vi "Lidar Control Error.vi"(0 "Lidar Motor Control":T1={"Reset Encoder"=FALSE, "Motor Enable"=FALSE, "Choice of Control Type"=enum."Direct Voltage Control", "Choice of Oscillation"=enum."Oscillate Voltage", "Choice of Compensation"=enum."None", "Choice of Error"=enum."Gray Error", "Units of pi rad 18b (s-fxp-1)"={"Phi_B Set Point (pi rad)"=0.0, "Phi_A Set Point (pi rad)"=0.0, "Phi_Lidar Set Point (pi rad)"=0.0, "Phi_Lidar - Phi_A"=0.0, "Phi_mass-Phi_Lidar"=0.0, "Convert (enc) to (pi rad)"=0.0, "Oscillation Frequency (pi rad per 100KHz)"=0.0}, "Units of 18b (s-fxp-1) gain"={"Proportional Gain"=0.0, " Integral Gain"=0.0, "Oscillation Setpoint Amplitude"=0.0, "Gravity Compensation Gain"=0.0, "Phi_B Set Point (enc) pre-gain"=0.0, "Phi_B Set Point (pi rad) pre-gain"=0.0, "Phi_A Set Point (pi rad) pre-gain"=0.0, "Phi_Lidar Set Point (pi rad) pre-gain"=0.0, "Derivative Gain"=0.0, "Double Integral Gain"=0.0, "Second Derivative Gain"=0.0}, "Units of 20b s-fxp-5 Voltage"={"Oscillation Voltage Amplitude"=0.0, "Motor Voltage"=0.0}, "Units of encoder 32b uint"={"Phi_B Set Point (enc)"=0, "Lidar Encoder Cap"=0}, "Debug Args"=[FALSE, FALSE, FALSE, FALSE, FALSE, FALSE, FALSE, FALSE, FALSE, FALSE, FALSE, FALSE, FALSE, FALSE, FALSE, FALSE, FALSE, FALSE, FALSE, FALSE], "Units of 8b int gain exponents"={"Proportional Gain"=0, " Integral Gain"=0, "Oscillation Setpoint Amplitude"=0, "Gravity Compensation Gain"=0, "Phi_B Set Point (enc) pre-gain"=0, "Phi_B Set Point (pi rad) pre-gain"=0, "Phi_A Set Point (pi rad) pre-gain"=0, "Phi_Lidar Set Point (pi rad) pre-gain"=0, "Derivative Gain"=0, "Double Integral Gain"=0, "Second Derivative Gain"=0}, "6b (u-fxp-6)"={"Size of Integrator"=0.0, "Size of IIntigrator"=0.0, "Size of Differentiator"=0.0, "Size of DDifferentiator"=0.0}} {"Units of 20b s-fxp-5 Voltage"."Motor Voltage" format="%.17g"}) -> ()   [LabVIEW 2009]
uses:
  Strict Lidar Motor Control Cluster.ctl
  [Debug] Global.vi
  Motor Output Global.vi
  Motor Control Global.vi
panel:
  out "I Error":fxp<+/-,18,1> format="%.18g"
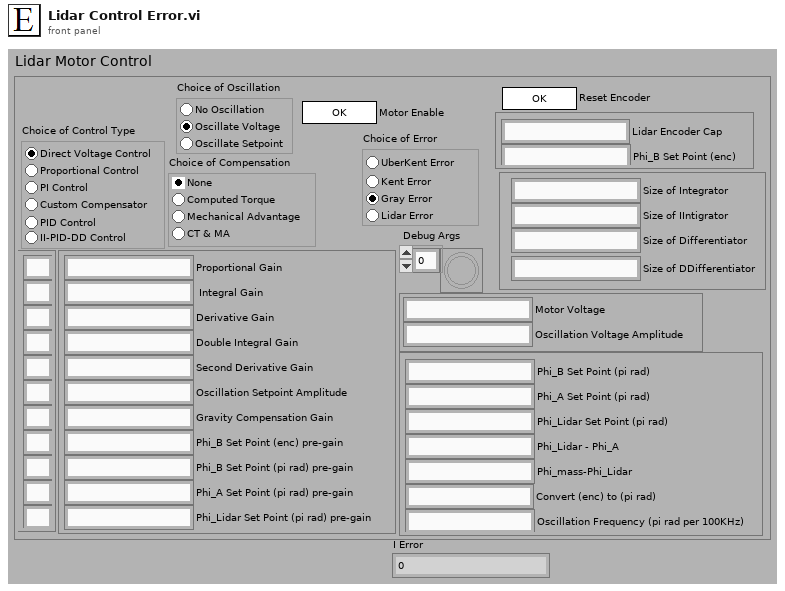
[diagram p1: front panel]
types:
  T1 = typedef "Strict Lidar Motor Control Cluster.ctl" = cluster{"Reset Encoder":bool, "Motor Enable":bool, "Choice of Control Type":enum32{"Direct Voltage Control", "Proportional Control", "PI Control", "Custom Compensator", "PID Control", "II-PID-DD Control"}, "Choice of Oscillation":enum32{"Oscillate Voltage", "Oscillate Setpoint", "No Oscillation"}, "Choice of Compensation":enum32{"None", "Computed Torque", "Mechanical Advantage", "CT & MA "}, "Choice of Error":enum32{"Gray Error", "Lidar Error", "Kent Error", "UberKent Error"}, "Units of pi rad 18b (s-fxp-1)":cluster{"Phi_B Set Point (pi rad)":fxp<+/-,18,1>, "Phi_A Set Point (pi rad)":fxp<+/-,18,1>, "Phi_Lidar Set Point (pi rad)":fxp<+/-,18,1>, "Phi_Lidar - Phi_A":fxp<+/-,18,1>, "Phi_mass-Phi_Lidar":fxp<+/-,18,1>, "Convert (enc) to (pi rad)":fxp<+/-,18,1>, "Oscillation Frequency (pi rad per 100KHz)":fxp<+/-,18,1>}, "Units of 18b (s-fxp-1) gain":cluster{"Proportional Gain":fxp<+/-,18,1>, " Integral Gain":fxp<+/-,18,1>, "Oscillation Setpoint Amplitude":fxp<+/-,18,1>, "Gravity Compensation Gain":fxp<+/-,18,1>, "Phi_B Set Point (enc) pre-gain":fxp<+/-,18,1>, "Phi_B Set Point (pi rad) pre-gain":fxp<+/-,18,1>, "Phi_A Set Point (pi rad) pre-gain":fxp<+/-,18,1>, "Phi_Lidar Set Point (pi rad) pre-gain":fxp<+/-,18,1>, "Derivative Gain":fxp<+/-,18,1>, "Double Integral Gain":fxp<+/-,18,1>, "Second Derivative Gain":fxp<+/-,18,1>}, "Units of 20b s-fxp-5 Voltage":cluster{"Oscillation Voltage Amplitude":fxp<+/-,20,5>, "Motor Voltage":fxp<+/-,20,5>}, "Units of encoder 32b uint":cluster{"Phi_B Set Point (enc)":i32, "Lidar Encoder Cap":i32}, "Debug Args":bool[], "Units of 8b int gain exponents":cluster{"Proportional Gain":i8, " Integral Gain":i8, "Oscillation Setpoint Amplitude":i8, "Gravity Compensation Gain":i8, "Phi_B Set Point (enc) pre-gain":i8, "Phi_B Set Point (pi rad) pre-gain":i8, "Phi_A Set Point (pi rad) pre-gain":i8, "Phi_Lidar Set Point (pi rad) pre-gain":i8, "Derivative Gain":i8, "Double Integral Gain":i8, "Second Derivative Gain":i8}, "6b (u-fxp-6)":cluster{"Size of Integrator":fxp<+,6,6>, "Size of IIntigrator":fxp<+,6,6>, "Size of Differentiator":fxp<+,6,6>, "Size of DDifferentiator":fxp<+,6,6>}}
  T2 = enum32{"Gray Error", "Lidar Error", "Kent Error", "UberKent Error"}
  T3 = cluster{"Debug Args[0]":bool, "Debug Args[1]":bool, "Debug Args[2]":bool, "Debug Args[3]":bool, "Debug Args[4]":bool, "Debug Args[5]":bool, "Debug Args[6]":bool, "Debug Args[7]":bool, "Debug Args[8]":bool}
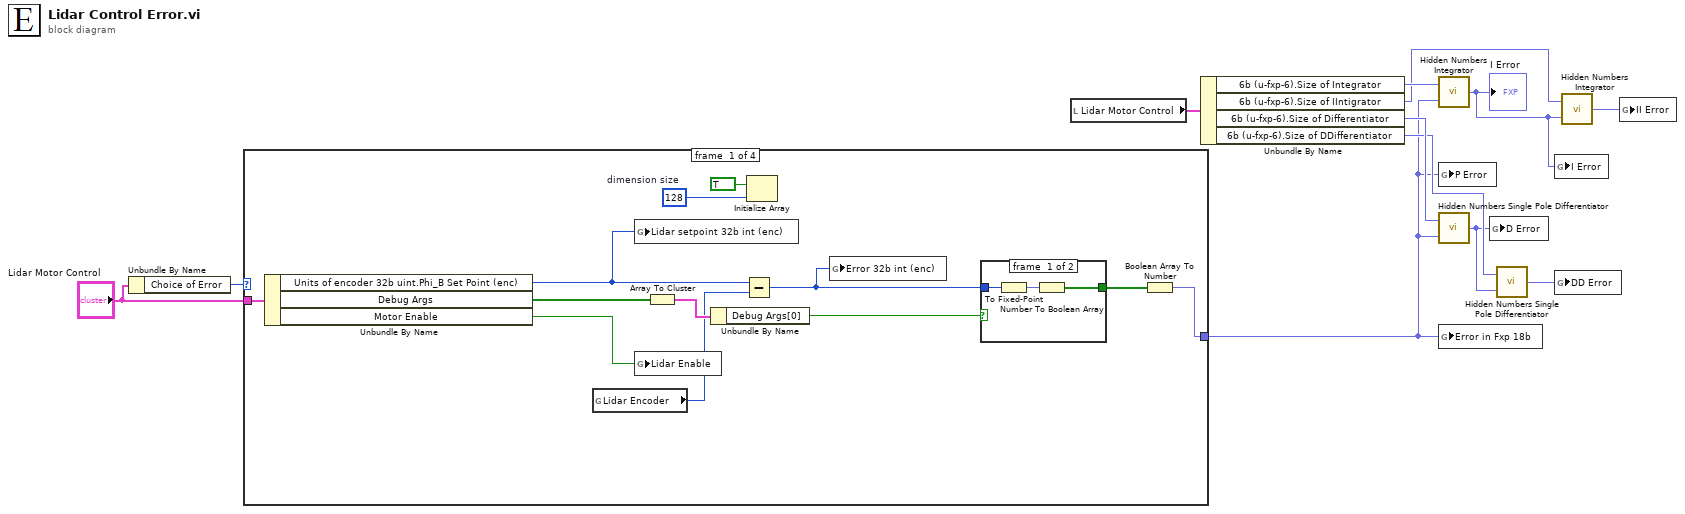
[diagram p0: block diagram]
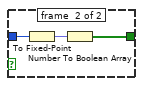
[diagram p2: hidden frame]
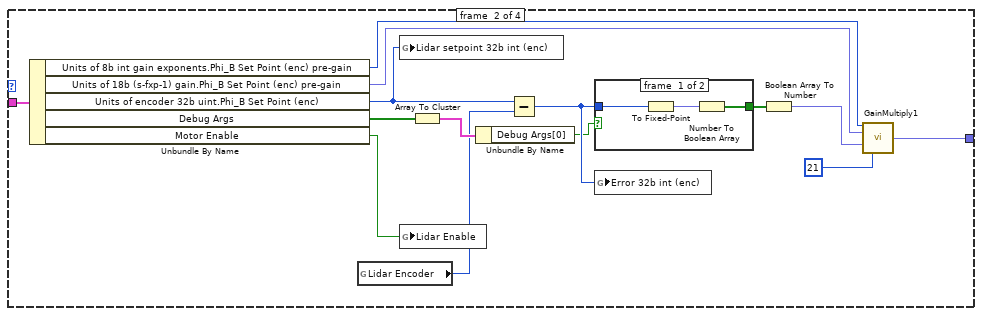
[diagram p3: hidden frame]
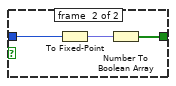
[diagram p4: hidden frame]
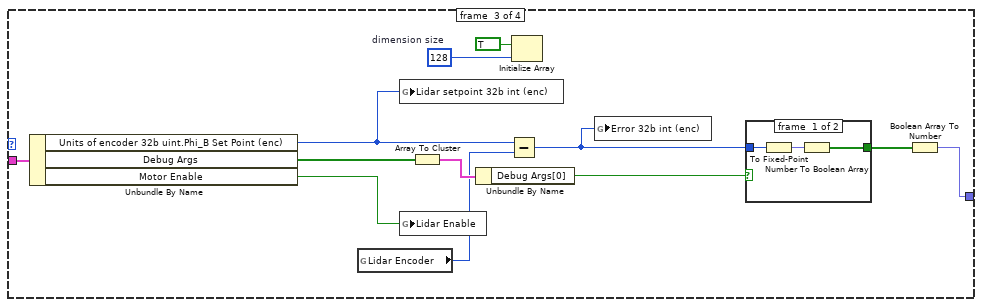
[diagram p5: hidden frame]
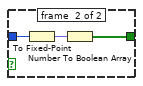
[diagram p6: hidden frame]
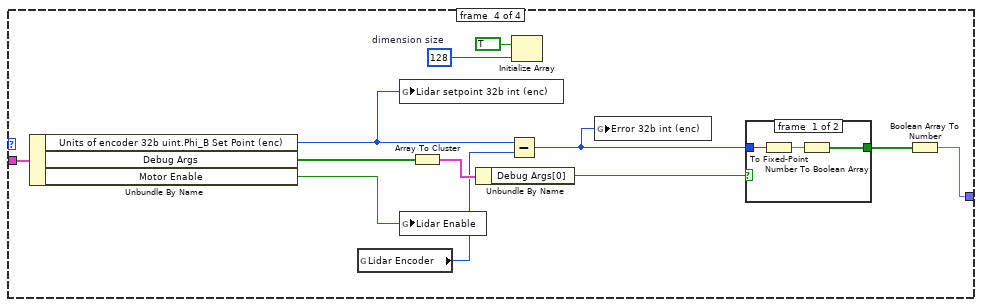
[diagram p7: hidden frame]
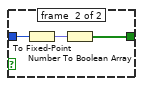
[diagram p8: hidden frame]
diagram:
  n1 = Unbundle By Name("Lidar Motor Control") -> ("Choice of Error"=w12:T2)
  n2 = case shown="\"UberKent Error\"" w12 {
    tunnel: [w15 w35 w53 w71] -> w3
    tunnel: "Lidar Motor Control" -> [w16 w36 w54 w72]
    frame #0 {
      w13 = 128  # dimension size
      n3 = Unbundle By Name(w16) -> ("Units of encoder 32b uint.Phi_B Set Point (enc)"=w23:i32, "Debug Args"=w19:bool[], "Motor Enable"=w21:bool)
      n4 = global read "Motor Control Global.vi" "Lidar Encoder"() -> (w18:i32)
      n5 = global write "[Debug] Global.vi" "Lidar setpoint 32b int (enc)"(w23) -> ()
      n6 = global write "Motor Output Global.vi" "Lidar Enable"(w21) -> ()
      n7 = Array To Cluster(array=w19) -> (cluster=w20:T3)
      n8 = Unbundle By Name(w20) -> ("Debug Args[0]"=w17:bool)
      n9 = Subtract(x=w23, y=w18) -> (x-y=w22:i32)
      n10 = Initialize Array(TRUE, w13) -> ()  [unwired: 1 out]
      n11 = global write "[Debug] Global.vi" "Error 32b int (enc)"(w22) -> ()
      n12 = case shown="False" w17 {
        tunnel: [w26 w30] -> w24
        tunnel: w22 -> [w25 w28]
        frame #0 {
          n13 = To Fixed-Point(number=w25) -> (fixed-point=w27:fxp<+/-,18,18>)  [unwired: 1 in]
          n14 = Number To Boolean Array(number=w27) -> (Boolean array=w26:bool[])
        }
        frame #1 {
          n15 = To Fixed-Point(number=w28) -> (fixed-point=w29:fxp<+/-,18,22>)  [unwired: 1 in]
          n16 = Number To Boolean Array(number=w29) -> (Boolean array=w30:bool[])
        }
      }
      n17 = Boolean Array To Number(Boolean array=w24) -> (number=w15:fxp<+/-,18,1>)
    }
    frame #1 {
      n18 = Unbundle By Name(w36) -> ("Units of 8b int gain exponents.Phi_B Set Point (enc) pre-gain"=w32:i8, "Units of 18b (s-fxp-1) gain.Phi_B Set Point (enc) pre-gain"=w33:fxp<+/-,18,1>, "Units of encoder 32b uint.Phi_B Set Point (enc)"=w43:i32, "Debug Args"=w39:bool[], "Motor Enable"=w41:bool)
      n19 = global read "Motor Control Global.vi" "Lidar Encoder"() -> (w38:i32)
      n20 = global write "[Debug] Global.vi" "Lidar setpoint 32b int (enc)"(w43) -> ()
      n21 = global write "Motor Output Global.vi" "Lidar Enable"(w41) -> ()
      n22 = Array To Cluster(array=w39) -> (cluster=w40:T3)
      n23 = Unbundle By Name(w40) -> ("Debug Args[0]"=w37:bool)
      n24 = Subtract(x=w43, y=w38) -> (x-y=w42:i32)
      n25 = case shown="False" w37 {
        tunnel: [w46 w50] -> w44
        tunnel: w42 -> [w45 w48]
        frame #0 {
          n26 = To Fixed-Point(number=w45) -> (fixed-point=w47:fxp<+/-,18,18>)  [unwired: 1 in]
          n27 = Number To Boolean Array(number=w47) -> (Boolean array=w46:bool[])
        }
        frame #1 {
          n28 = To Fixed-Point(number=w48) -> (fixed-point=w49:fxp<+/-,18,22>)  [unwired: 1 in]
          n29 = Number To Boolean Array(number=w49) -> (Boolean array=w50:bool[])
        }
      }
      n30 = global write "[Debug] Global.vi" "Error 32b int (enc)"(w42) -> ()
      n31 = Boolean Array To Number(Boolean array=w44) -> (number=w34:fxp<+/-,18,1>)
      n32 = call "GainMultiply1.vi"("Gain Exponent"=w32, "Gain"=w33, "Input"=w34, "Unique 8b identifier"=u8 21) -> ("Output"=w35:fxp<+/-,18,1>)  [unwired: 9 in, 2 out]
    }
    frame #2 {
      w51 = 128  # dimension size
      n33 = Unbundle By Name(w54) -> ("Units of encoder 32b uint.Phi_B Set Point (enc)"=w61:i32, "Debug Args"=w57:bool[], "Motor Enable"=w59:bool)
      n34 = global read "Motor Control Global.vi" "Lidar Encoder"() -> (w56:i32)
      n35 = global write "[Debug] Global.vi" "Lidar setpoint 32b int (enc)"(w61) -> ()
      n36 = global write "Motor Output Global.vi" "Lidar Enable"(w59) -> ()
      n37 = Array To Cluster(array=w57) -> (cluster=w58:T3)
      n38 = Unbundle By Name(w58) -> ("Debug Args[0]"=w55:bool)
      n39 = Subtract(x=w61, y=w56) -> (x-y=w60:i32)
      n40 = Initialize Array(TRUE, w51) -> ()  [unwired: 1 out]
      n41 = global write "[Debug] Global.vi" "Error 32b int (enc)"(w60) -> ()
      n42 = case shown="False" w55 {
        tunnel: [w64 w68] -> w62
        tunnel: w60 -> [w63 w66]
        frame #0 {
          n43 = To Fixed-Point(number=w63) -> (fixed-point=w65:fxp<+/-,18,18>)  [unwired: 1 in]
          n44 = Number To Boolean Array(number=w65) -> (Boolean array=w64:bool[])
        }
        frame #1 {
          n45 = To Fixed-Point(number=w66) -> (fixed-point=w67:fxp<+/-,18,22>)  [unwired: 1 in]
          n46 = Number To Boolean Array(number=w67) -> (Boolean array=w68:bool[])
        }
      }
      n47 = Boolean Array To Number(Boolean array=w62) -> (number=w53:fxp<+/-,18,1>)
    }
    frame #3 {
      w69 = 128  # dimension size
      n48 = Unbundle By Name(w72) -> ("Units of encoder 32b uint.Phi_B Set Point (enc)"=w79:i32, "Debug Args"=w75:bool[], "Motor Enable"=w77:bool)
      n49 = global read "Motor Control Global.vi" "Lidar Encoder"() -> (w74:i32)
      n50 = global write "[Debug] Global.vi" "Lidar setpoint 32b int (enc)"(w79) -> ()
      n51 = global write "Motor Output Global.vi" "Lidar Enable"(w77) -> ()
      n52 = Array To Cluster(array=w75) -> (cluster=w76:T3)
      n53 = Unbundle By Name(w76) -> ("Debug Args[0]"=w73:bool)
      n54 = Subtract(x=w79, y=w74) -> (x-y=w78:i32)
      n55 = Initialize Array(TRUE, w69) -> ()  [unwired: 1 out]
      n56 = global write "[Debug] Global.vi" "Error 32b int (enc)"(w78) -> ()
      n57 = case shown="False" w73 {
        tunnel: [w82 w86] -> w80
        tunnel: w78 -> [w81 w84]
        frame #0 {
          n58 = To Fixed-Point(number=w81) -> (fixed-point=w83:fxp<+/-,18,18>)  [unwired: 1 in]
          n59 = Number To Boolean Array(number=w83) -> (Boolean array=w82:bool[])
        }
        frame #1 {
          n60 = To Fixed-Point(number=w84) -> (fixed-point=w85:fxp<+/-,18,22>)  [unwired: 1 in]
          n61 = Number To Boolean Array(number=w85) -> (Boolean array=w86:bool[])
        }
      }
      n62 = Boolean Array To Number(Boolean array=w80) -> (number=w71:fxp<+/-,18,1>)
    }
  }
  n63 = local read "Lidar Motor Control"() -> (w10:T1)
  n64 = Unbundle By Name(w10) -> ("6b (u-fxp-6).Size of Integrator"=w9:fxp<+,6,6>, "6b (u-fxp-6).Size of IIntigrator"=w8:fxp<+,6,6>, "6b (u-fxp-6).Size of Differentiator"=w5:fxp<+,6,6>, "6b (u-fxp-6).Size of DDifferentiator"=w4:fxp<+,6,6>)
  n65 = call "Hidden Numbers Integrator.vi"("Integrand"=w3, "Size of Integrator"=w9) -> ("18b (s-fxp-1) out"=w7:fxp<+/-,18,1>)
  "I Error" <- w7
  n66 = global write "[Debug] Global.vi" "P Error"(w3) -> ()
  n67 = call "Hidden Numbers Single Pole Differentiator.vi"("18b (s-fxp-1) Input (A)"=w3, "N"=w5) -> ("18b (s-fxp-1) out"=w2:fxp<+/-,18,1>)
  n68 = global write "[Debug] Global.vi" "Error in Fxp 18b"(w3) -> ()
  n69 = global write "[Debug] Global.vi" "D Error"(w2) -> ()
  n70 = call "Hidden Numbers Single Pole Differentiator.vi"("18b (s-fxp-1) Input (A)"=w2, "N"=w4) -> ("18b (s-fxp-1) out"=w1:fxp<+/-,18,1>)
  n71 = global write "[Debug] Global.vi" "I Error"(w7) -> ()
  n72 = global write "[Debug] Global.vi" "DD Error"(w1) -> ()
  n73 = call "Hidden Numbers Integrator.vi"("Integrand"=w7, "Size of Integrator"=w8) -> ("18b (s-fxp-1) out"=w6:fxp<+/-,18,1>)
  n74 = global write "[Debug] Global.vi" "II Error"(w6) -> ()
